vi "Example Callback.vi"() -> ()   [LabVIEW 2010]
uses:
  C:/tf/play/labview/Tinkerforge.dll
panel:
  out "touch state":string
  in  "stop":bool
  in  "uid":string="fdsg"
  in  "port":i32=4223
  in  "host":string="localhost"
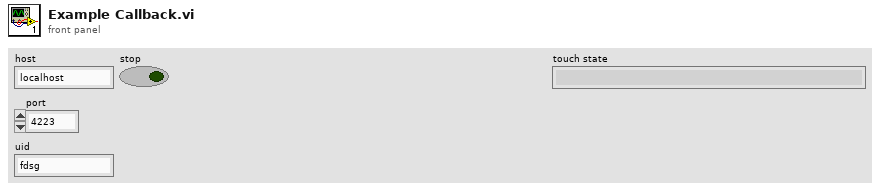
[diagram p1: front panel]
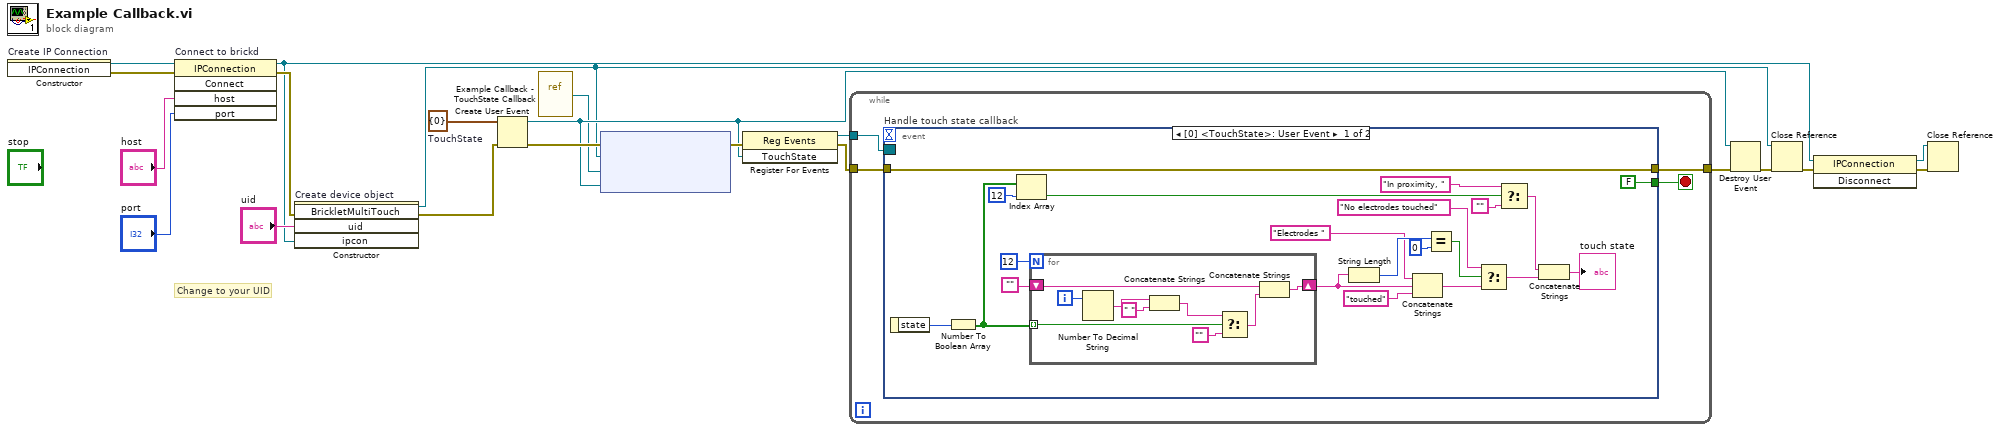
[diagram p0: block diagram]
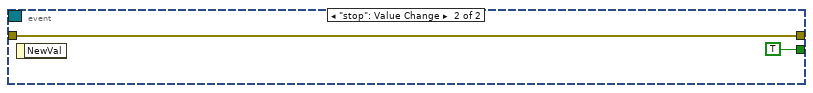
[diagram p2: hidden frame]
diagram:
  w5 = cluster{"state":i32} {"state"=0}  # TouchState
  # "Change to your UID"
  n1 = constructor on="Create IP Connection" class="IPConnection"() -> (reference out=w21:refnum<k24>, error out=w4:errorcluster)  [unwired: 3 in, 1 out]
  n2 = invoke on="Connect to brickd" class="IPConnection" method="Connect"(reference=w21, error in=w4, "host"="host", "port"="port") -> (reference out=w14:refnum<k24>, error out=w17:errorcluster)  [unwired: 1 in, 3 out]
  n3 = constructor on="Create device object" class="BrickletMultiTouch"(error in=w17, "uid"="uid", "ipcon"=w14) -> (reference out=w2:refnum<k24>, error out=w3:errorcluster)  [unwired: 2 in, 3 out]
  n4 = Create User Event(user event datatype=w5, error in=w3) -> (user event=w7:refnum<user-event>, error out=w12:errorcluster)
  n5 = vi-ref "Example Callback - TouchState Callback.vi"() -> ("vi reference"=w1:refnum<vi>)
  n6 = node ("Register Event Callback")(w12, w2, w1, w7) -> (w11:errorcluster)  [unwired: 1 in, 1 out]
  n7 = register-events(error in=w11, w7) -> (reference out=w10:refnum<event-registration>, error out=w8:errorcluster)  [unwired: 1 in]
  n8 = while {
    tunnel: w10 -> [w25]
    tunnel: [w24] -> w9
    tunnel: w8 -> [w23]
    stop <- w22 stop-if-true
    n9 = event "Handle touch state callback" shown="[0] <TouchState>: User Event" {
      selector: w25 -> [_ _]
      dyn-events: _ -> [_ _]
      timeout: _ -> [_ _]
      tunnel: [w46 w56] -> w24
      tunnel: w23 -> [w46 w56]
      tunnel: [FALSE TRUE] -> w22
      event User Event {
        n10 = event-data() -> ("state"=w27:i32)  [unwired: 1 in]
        n11 = Number To Boolean Array(number=w27) -> (Boolean array=w40:bool[])
        n12 = Index Array(array=w40, index=12) -> (element=w41:bool)
        n13 = for {
          N: 12 -> [_]
          tunnel: w40 -> [w55] mode=indexing
          shift-right: [w51] -> w33
          shift-left: "" -> [w52]
          i -> [w50]
          n14 = Number To Decimal String(number=w50) -> (decimal integer string=w48:string)  [unwired: 1 in]
          n15 = Concatenate Strings(w48, " " ("string")) -> (w49:string)
          n16 = Select(t=w49, s=w55, f="") -> (s? t:f=w53:string)
          n17 = Concatenate Strings(w52, w53) -> (w51:string)
        }
        n18 = String Length(string=w33) -> (length=w37:i32)
        n19 = Concatenate Strings("Electrodes " ("string"), w33, "touched" ("string")) -> (w32:string)
        n20 = Equal?(x=w37, y=0) -> (x = y?=w35:bool)
        n21 = Select(t="No electrodes touched", s=w35, f=w32) -> (s? t:f=w28:string)
        n22 = Select(t="In proximity, ", s=w41, f="") -> (s? t:f=w29:string)
        n23 = Concatenate Strings(w29, w28) -> (→"touch state":string)
      }
      event "stop": Value Change {
        n24 = event-data() -> ()  [unwired: 1 in, 1 out]
      }
    }
  }
  n25 = Destroy User Event(user event=w7, error in=w9) -> (error out=w6:errorcluster)
  n26 = Close Reference(reference=w2, error in (no error)=w6) -> (error out=w16:errorcluster)
  n27 = invoke class="IPConnection" method="Disconnect"(reference=w14, error in=w16) -> (reference out=w13:refnum<k24>, error out=w15:errorcluster)  [unwired: 1 in, 1 out]
  n28 = Close Reference(reference=w13, error in (no error)=w15) -> ()  [unwired: 1 out]
